vi "SaveDataSGLFast.vi"(7 "Header In":T1 {"Compression Parameters"."% taper" min=50 max=1000 format="%.2f"; "Compression Parameters"."F2 (MHz)" format="%.3f"; "Compression Parameters"."F1 (MHz)" format="%.3f"; "Scan Settings"."prf (kHz)" format="%.2f"; "Therapy Parameters"."Therapy amplitude (mV)" min=50 max=1000 format="%.2f"; "Therapy Parameters"."Time on (s)" format="%.3f"; "Therapy Parameters"."Theraputic Freq (MHz)" format="%.3f"; "Patient Info"."Race" items=["Am Ind or Alaska", "Asian", "Hawaiian, Pac Isl", "Black or Afr Amer", "White", "more than one race", "unknown"]; "Patient Info"."Ethnicty 2" items=["Hispanic", "Non-Hispanic", "unknown"]; "Patient Info"."LOS" items=["1", "2", "3", "4", "5"]; "Patient Info"."PSA" format="%.1f"; "Scan Info"."delay" format="%.2f"; "Scan Info"."pivot distance" format="%.2f"; "Scan Info"."sector scan angle" format="%.2f"; "Tranducer Info"."bandwidth" format="%.2f"; "Tranducer Info"."center freq" format="%.2f"; "Tranducer Info"."start freq" format="%.2f"}, 8 "error in (no error)":errorcluster, 9 "Save?":bool, 10 "Data Array":sgl[][](array[numeric]), 11 "File Name and Path":path) -> (0 "error out":errorcluster)   [LabVIEW 2022 SP3]
uses:
  Header.ctl
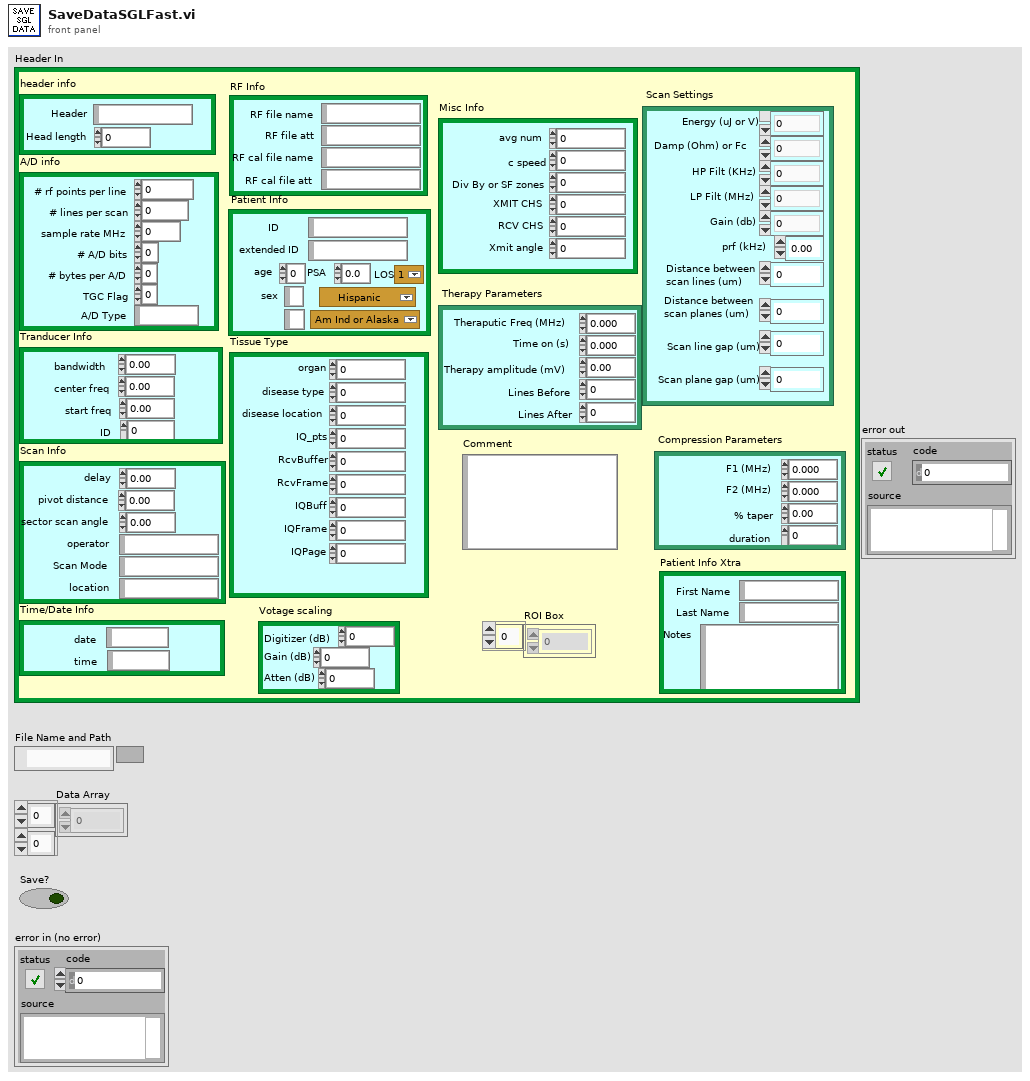
[diagram p1: front panel]
types:
  T1 = typedef "Header.ctl" = cluster{"header info":cluster{"Header":string, "Head length":i16}, "A/D info":cluster{"# rf points per line":u16, "# lines per scan":u16, "sample rate MHz":u16, "# A/D bits":i16, "# bytes per A/D":u16, "TGC Flag":u16, "A/D Type":string}, "Tranducer Info":cluster{"bandwidth":sgl, "center freq":sgl, "start freq":sgl, "ID":i32}, "Scan Info":cluster{"delay":sgl, "pivot distance":sgl, "sector scan angle":sgl, "operator":string, "Scan Mode":string, "location":string}, "Time/Date Info":cluster{"date":string, "time":string}, "RF Info":cluster{"RF file name":string, "RF file att":string, "RF cal file name":string, "RF cal file att":string}, "Patient Info":cluster{"ID":string, "extended ID":string, "age":u16, "sex":string, "previously\nscanned":string, "PSA":sgl, "LOS":u8, "Ethnicty 2":u8, "Race":u8}, "Tissue Type":cluster{"organ":i16, "disease type":i16, "disease location":i16, "IQ_pts":u16, "RcvBuffer":u8, "RcvFrame":u16, "IQBuff":u8, "IQFrame":u16, "IQPage":u8}, "Votage scaling":cluster{"Digitizer (dB)":sgl, "Gain (dB)":sgl, "Atten (dB)":sgl}, "Comment":string, "Misc Info":cluster{"avg num":u16, "c speed":i16, "Div By or SF zones":i16, "XMIT CHS":u8, "RCV CHS":u8, "Xmit angle":sgl}, "Therapy Parameters":cluster{"Theraputic Freq (MHz)":sgl, "Time on (s)":sgl, "Therapy amplitude (mV)":sgl, "Lines Before":u16, "Lines After":u16}, "Scan Settings":cluster{"Energy (uJ or V)":u8, "Damp (Ohm) or Fc":u8, "HP Filt (KHz)":u8, "LP Filt (MHz)":u8, "Gain (db)":u8, "prf (kHz)":sgl, "Distance between\nscan lines (um)":u16, "Distance between\nscan planes (um)":u16, "Scan line gap (um)":sgl, "Scan plane gap (um)":sgl}, "Compression Parameters":cluster{"F1 (MHz)":sgl, "F2 (MHz)":sgl, "% taper":sgl, "duration":sgl}, "Patient Info Xtra":cluster{"First Name":string, "Last Name":string, "Notes":string}, "ROI Box":u16[]}
  T2 = enum16{"big-endian, network order", "native, host order", "little-endian"}
  T3 = enum16{"open", "replace", "create", "open or create", "replace or create", "replace or create with confirmation"}
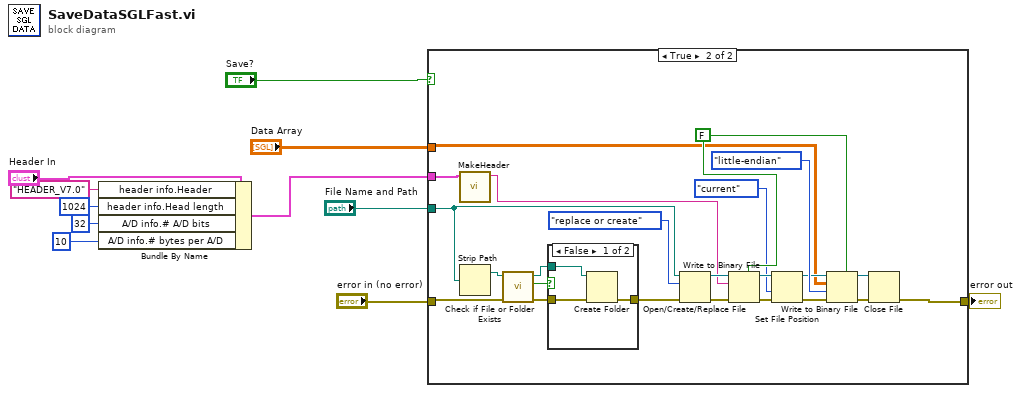
[diagram p0: block diagram]
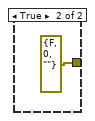
[diagram p3: hidden frame]
diagram:
  n1 = Bundle By Name(cluster="Header In", "header info.Header"="HEADER_V7.0", "header info.Head length"=i16 1024, "A/D info.# A/D bits"=i16 32, "A/D info.# bytes per A/D"=u16 10) -> (w3:T1)
  n2 = case shown="True" "Save?" {
    tunnel: w3 -> [_ w35]
    tunnel: "File Name and Path" -> [_ w15]
    tunnel: "Data Array" -> [_ w21]
    tunnel: "error in (no error)" -> [w12 w14]
    tunnel: [w12 w20] -> w8
    frame False {
    }
    frame True {
      w33 = FALSE ("prepend array or string size? (T)")
      n3 = call "MakeHeader.vi"("Header In"=w35) -> ("Header String"=w22:string)  [unwired: 6 out]
      n4 = Strip Path(path=w15) -> (stripped path=w16:path)  [unwired: 1 out]
      n5 = call <vilib>:"Check if File or Folder Exists.vi"("error in (no error)"=w14, "path"=w16) -> ("error out"=w19:errorcluster, "file or folder exists?"=w17:bool, "dup path"=w18:path)  [unwired: 7 in]
      n6 = case shown="False" w17 {
        tunnel: w19 -> [w38 _]
        tunnel: w18 -> [w37 _]
        tunnel: [w36 errorcluster {"status"=FALSE, "code"=0, "source"=""} ("error out")] -> w13
        frame False {
          n7 = Create Folder(path (use dialog)=w37, error in=w38) -> (error out=w36:errorcluster)  [unwired: 1 in, 2 out]
        }
        frame True {
        }
      }
      n8 = Open/Create/Replace File(file path (use dialog)=w15, error in=w13, operation (0:open)=T3."replace or create") -> (refnum out=w29:refnum<file>, error out=w30:errorcluster)  [unwired: 4 out]
      n9 = Write to Binary File(file (use dialog)=w29, data=w22, error in=w30, 5:w33) -> (refnum out=w27:refnum<file>, error out=w28:errorcluster)  [unwired: 3 out]
      n10 = Set File Position(refnum=w27, from (0:start)=enum16{"start", "end", "current"}."current" ("pos mode (0:2)"), error in=w28) -> (refnum out=w31:refnum<file>, error out=w32:errorcluster)  [unwired: 1 out]
      n11 = Write to Binary File(file (use dialog)=w31, data=w21, error in=w32, 5:w33, 9:T2."little-endian" ("byte order (0:big-endian, network order)")) -> (refnum out=w25:refnum<file>, error out=w24:errorcluster)  [unwired: 2 out]
      n12 = Close File(refnum=w25, error in=w24) -> (error out=w20:errorcluster)  [unwired: 1 out]
    }
  }
  "error out" <- w8
